vi "Main_Test.vi"() -> ()   [LabVIEW 2026]
panel:
  in  "VISA resource name":refnum<visa-resource-name>
  out "raw response":string
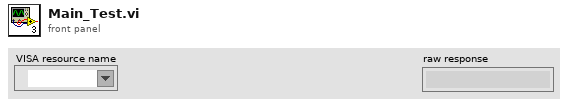
[diagram p1: front panel]
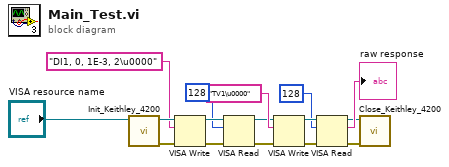
[diagram p0: block diagram]
diagram:
  n1 = call "Init_Keithley_4200.vi"("VISA resource name"="VISA resource name") -> ("error out"=w15:errorcluster, "VISA resource name out"=w16:refnum<visa-resource-name>)  [unwired: 9 in]
  n2 = VISA Write(VISA resource name=w16, write buffer="DI1, 0, 1E-3, 2\u0000", error in (no error)=w15) -> (VISA resource name out=w5:refnum<visa-resource-name>, error out=w4:errorcluster)  [unwired: 1 out]
  n3 = VISA Read(VISA resource name=w5, byte count=u32 128, error in (no error)=w4) -> (VISA resource name out=w3:refnum<visa-resource-name>, error out=w2:errorcluster)  [unwired: 2 out]
  n4 = VISA Write(VISA resource name=w3, write buffer="TV1\u0000", error in (no error)=w2) -> (VISA resource name out=w14:refnum<visa-resource-name>, error out=w13:errorcluster)  [unwired: 1 out]
  n5 = VISA Read(VISA resource name=w14, byte count=u32 128, error in (no error)=w13) -> (VISA resource name out=w7:refnum<visa-resource-name>, read buffer=→"raw response":string, error out=w12:errorcluster)  [unwired: 1 out]
  n6 = call "Close_Keithley_4200.vi"("error in (no error)"=w12, "VISA resource name"=w7) -> ()  [unwired: 9 in, 1 out]
